vi "Get Picture.vi"(8 "error in (no error)":errorcluster, 11 "Battery Stack in":refnum<class "Battery Stack.lvclass">) -> (0 "error out":errorcluster, 2 "Picture":picture, 3 "Battery Stack out":refnum<class "Battery Stack.lvclass">)   [LabVIEW 2020, in "Battery Stack.lvclass"]
uses:
  Battery Stack.lvclass
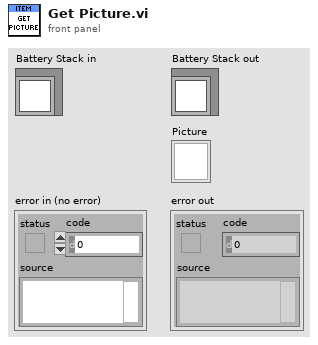
[diagram p1: front panel]
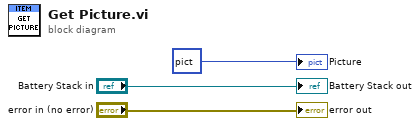
[diagram p0: block diagram]
diagram:
  "error out" <- "error in (no error)"
  "Battery Stack out" <- "Battery Stack in"
  "Picture" <- picture bytes[3230] ("new picture")
